vi "DriveMotors.vi"(8 "error in":errorcluster, 10 "Right Value":dbl, 11 "Left Value":dbl) -> (0 "error out":errorcluster)   [LabVIEW 2016]
uses:
  <vilib>/Rock Robotics/WPI/Utilities/WPI_GetSetVariantRefNum.vi
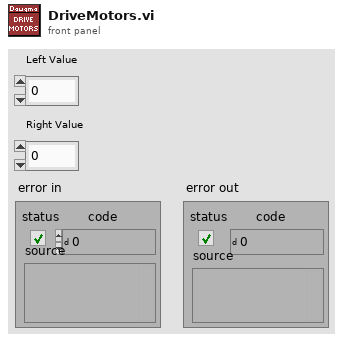
[diagram p1: front panel]
types:
  T1 = typedef "WPI_RobotDriveDevRef.ctl" = cluster{"DevStatus":errorcluster, "Motors[]":T2[], "Square Inputs":bool, "Max Output":dbl}
  T2 = typedef "WPI_MotorControlDeviceRef.ctl" = cluster{"DeviceStatus":errorcluster, "Type":T3, "PWM":cluster{"PWM Channel":T4, "DeadBand":T5}, "CAN":cluster{"Device Number":u8, "SetOutput VI Ref":variant, "GetOutput VI Ref":variant, "Enable VI Ref":variant, "Disable VI Ref":variant, "Data":variant}, "Invert":bool}
  T3 = typedef "WPI_MotorControlType.ctl" = enum16{"PWM", "CAN"}
  T4 = typedef "FPGA_DIOPWMChannel.ctl" = enum8{"PWM 0", "PWM 1", "PWM 2", "PWM 3", "PWM 4", "PWM 5", "PWM 6", "PWM 7", "PWM 8", "PWM 9", "PWM MXP 0", "PWM MXP 1", "PWM MXP 2", "PWM MXP 3", "PWM MXP 4", "PWM MXP 5", "PWM MXP 6", "PWM MXP 7", "PWM MXP 8", "PWM MXP 9", "Invalid"}
  T5 = typedef "WPI_PWMDeadband.ctl" = cluster{"Name":string, "maxPositivePwm":i32, "minPositivePwm":i32, "centerPwm":i32, "maxNegativePwm":i32, "minNegativePwm":i32, "angularRange":u16}
  T6 = cluster{"RobotDriveDevRef":T1, "RobotDriveDevRef":T1}
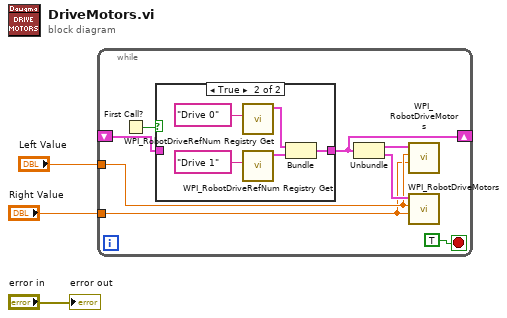
[diagram p0: block diagram]
diagram:
  n1 = while {
    shift-right: [w8] -> _
    shift-left: _ -> [w9]
    tunnel: "Left Value" -> [w5]
    tunnel: "Right Value" -> [w4]
    stop <- TRUE stop-if-true
    n2 = First Call?() -> (First Call?: T/F=w10:bool)
    n3 = case shown="True" w10 {
      tunnel: [w12 w17] -> w8
      tunnel: w9 -> [w12 _]
      frame False {
      }
      frame True {
        n4 = call <vilib>:"WPI_RobotDriveRefNum Registry Get.vi"("refnum name"="Drive 0") -> ("RobotDriveDevRef"=w13:T1)  [unwired: 9 in, 1 out]
        n5 = call <vilib>:"WPI_RobotDriveRefNum Registry Get.vi"("refnum name"="Drive 1") -> ("RobotDriveDevRef"=w14:T1)  [unwired: 9 in, 1 out]
        n6 = Bundle("RobotDriveDevRef"=w13, "RobotDriveDevRef"=w14) -> (w17:T6)  [unwired: 1 in]
      }
    }
    n7 = Unbundle(w8) -> ("RobotDriveDevRef"=w7:T1, "RobotDriveDevRef"=w6:T1)
    n8 = call <vilib>:"WPI_RobotDriveMotors.vi"("RightSpeed"=w4, "LeftSpeed"=w5, "RobotDriveDevRef"=w7) -> ()  [unwired: 6 in, 3 out]
    n9 = call <vilib>:"WPI_RobotDriveMotors.vi"("RightSpeed"=w4, "LeftSpeed"=w5, "RobotDriveDevRef"=w6) -> ()  [unwired: 6 in, 3 out]
  }
  "error out" <- "error in"
